vi "Is HexStr Content.vi"(11 "Content":string) -> (2 "hexStr":string, 3 "HexStr Content":bool)   [LabVIEW 2017, in "INI-Static-Variable-Support.lvlib"]
uses:
  INI-Static-Variable-Support.lvlib
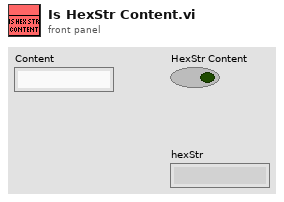
[diagram p1: front panel]
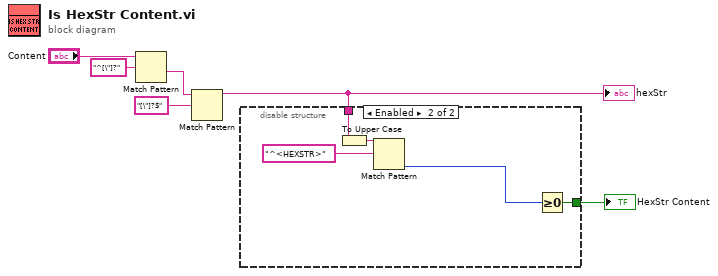
[diagram p0: block diagram]
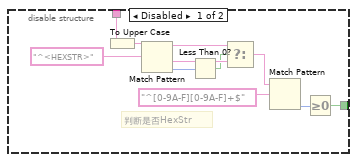
[diagram p2: hidden frame]
diagram:
  n1 = Match Pattern(string="Content", regular expression="^[\"]?") -> (after substring=w2:string)  [unwired: 1 in, 3 out]
  n2 = Match Pattern(string=w2, regular expression="[\"]?$") -> (before substring=w1:string)  [unwired: 1 in, 3 out]
  "hexStr" <- w1
  n3 = disable-structure shown="Enabled" {
    disable-tunnel: [w17 w22] -> w6
    disable-tunnel: w1 -> [w7 w19]
    frame Disabled {
      # "判断是否HexStr"
      n4 = To Upper Case(1:w7) -> (0:w13:string)
      n5 = Match Pattern(string=w13, regular expression="^<HEXSTR>") -> (before substring=w11:string, after substring=w10:string, offset past match=w12:i32)  [unwired: 1 in, 1 out]
      n6 = Less Than 0?(x=w12) -> (x < 0?=w9:bool)
      n7 = Select(t=w11, s=w9, f=w10) -> (s? t:f=w8:string)
      n8 = Match Pattern(string=w8, regular expression="^[0-9A-F][0-9A-F]+$") -> (offset past match=w15:i32)  [unwired: 1 in, 3 out]
      n9 = Greater Or Equal To 0?(x=w15) -> (x >= 0?=w17:bool)
    }
    frame Enabled {
      n10 = To Upper Case(1:w19) -> (0:w20:string)
      n11 = Match Pattern(string=w20, regular expression="^<HEXSTR>") -> (offset past match=w18:i32)  [unwired: 1 in, 3 out]
      n12 = Greater Or Equal To 0?(x=w18) -> (x >= 0?=w22:bool)
    }
  }
  "HexStr Content" <- w6
